vi "Riccati_DARE_Choose.vi"(8 "R":T1, 9 "Q":T1, 10 "B":T1, 11 "A":T1) -> (0 "error out":errorcluster, 1 "Error":bool, 2 "Iterations":i32, 3 "Answer":T1)   [LabVIEW 2019, in "Trajectory_Library.lvlib"]
doc: "Solves the discrete alegebraic Riccati equation.\n \nInput:\n - A -- System matrix.\n - B -- nput matrix.\n - Q -- State cost matrix.\n - R -- Input cost matrix.\n\nOutputs:\n Answer -- Solution of DARE.\n iterations -- Number of iterations\n error -- If TRUE, an error occured"
uses:
  <vilib>/Analysis/Matrix/Datatypes/RealMatrix.ctl
  Trajectory_Library.lvlib
  <vilib>/Analysis/Matrix/NI_Matrix.lvlib
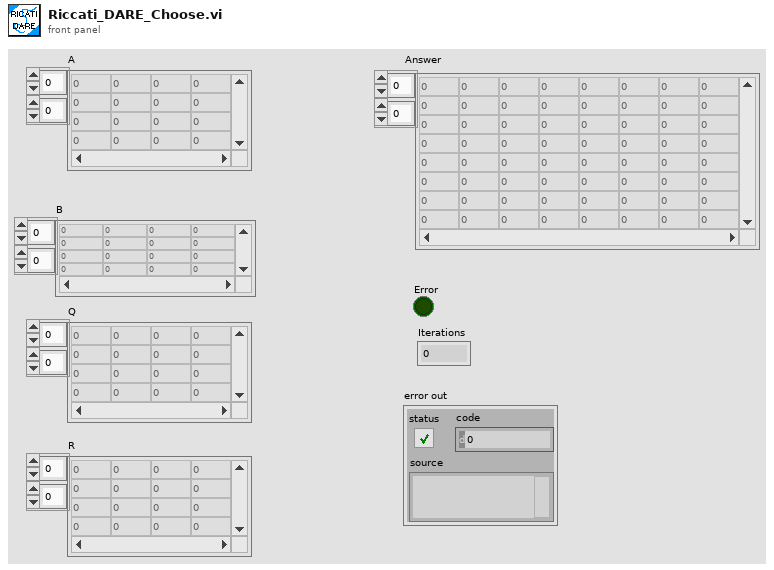
[diagram p1: front panel]
types:
  T1 = typedef "NI_Matrix.lvlib/RealMatrix.ctl" = dbl[][]
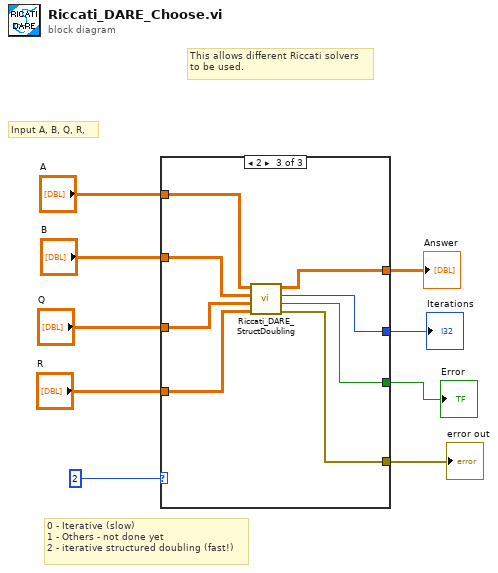
[diagram p0: block diagram]
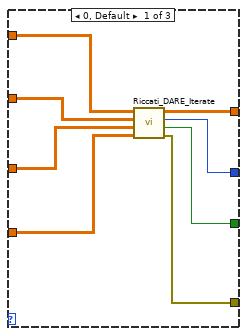
[diagram p2: hidden frame]
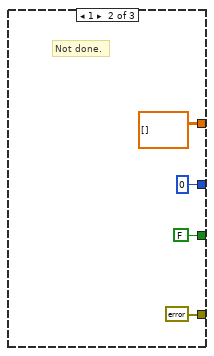
[diagram p3: hidden frame]
diagram:
  # "This allows different Riccati solvers\nto be used."
  # "0 - Iterative (slow)\n1 - Others - not done yet\n2 - iterative structured doubling (fast!)"
  # "Input A, B, Q, R,"
  n1 = case shown="2" 2 {
    tunnel: "A" -> [w17 _ w29]
    tunnel: "B" -> [w16 _ w28]
    tunnel: "Q" -> [w15 _ w27]
    tunnel: "R" -> [w14 _ w26]
    tunnel: [w13 T1 [] ("Answer") w25] -> w4
    tunnel: [w12 0 ("Iterations") w24] -> w3
    tunnel: [w11 FALSE ("Finished") w23] -> w2
    tunnel: [w10 errorcluster {"status"=FALSE, "code"=0, "source"=""} ("error out") w22] -> w1
    frame 0, Default {
      n2 = call "Riccati_DARE_Iterate.vi"("R"=w14, "Q"=w15, "B"=w16, "A"=w17) -> ("error out"=w10:errorcluster, "Error"=w11:bool, "Iterations"=w12:i32, "Answer"=w13:T1)  [unwired: 4 in]
    }
    frame 1 {
      # "Not done."
    }
    frame 2 {
      n3 = call "Riccati_DARE_StructDoubling.vi"("R"=w26, "Q"=w27, "B"=w28, "A"=w29) -> ("error out"=w22:errorcluster, "Error"=w23:bool, "Iterations"=w24:i32, "Answer"=w25:T1)  [unwired: 4 in]
    }
  }
  "Answer" <- w4
  "Iterations" <- w3
  "Error" <- w2
  "error out" <- w1
